vi "side_ir_microstep.vi"(0 "IN-OUT":enum16{"out", "in"}(ring), 1 "IR_L":dbl, 2 "IR_R":dbl, 5 "Step":i32, 7 "Stop Mode":string(combo), 9 "Delay":i32, 11 "logic_num":dbl, 12 "Zeta_B":i32, 13 "Zeta_F":i32) -> (4 "OZeta_b":i32, 6 "Ozeta_f":i32, 8 "Done":bool)   [LabVIEW 2017]
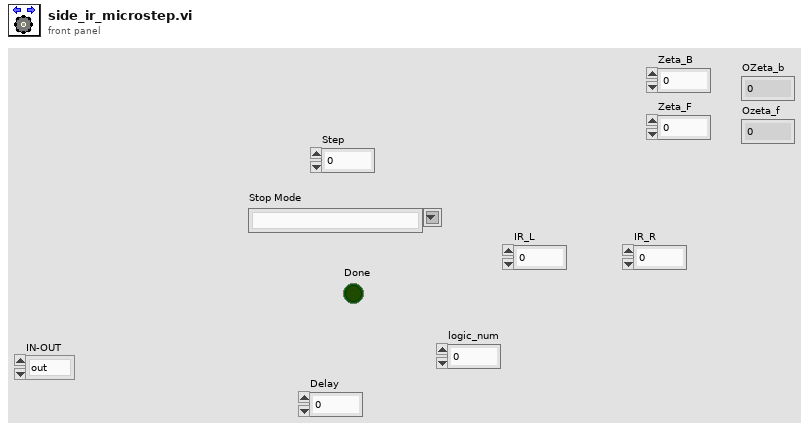
[diagram p1: front panel]
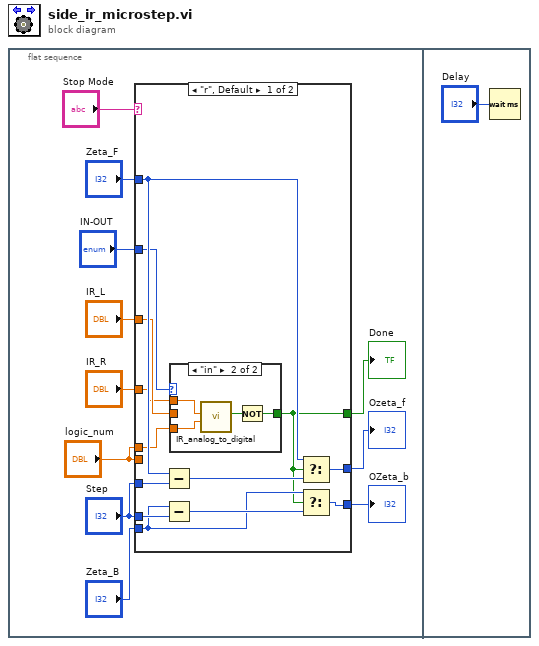
[diagram p0: block diagram]
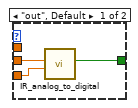
[diagram p2: hidden frame]
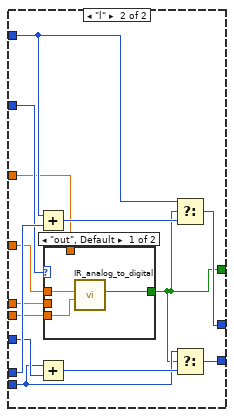
[diagram p3: hidden frame]
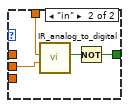
[diagram p4: hidden frame]
diagram:
  n1 = flat-sequence {
    frame #0 {
      n2 = case shown="\"r\", Default" "Stop Mode" {
        tunnel: "IR_L" -> [w15 w32]
        tunnel: "logic_num" -> [w14 w34]
        tunnel: [w19 w44] -> w5
        tunnel: [w20 w43] -> w4
        tunnel: [w13 w33] -> w9
        tunnel: "Zeta_B" -> [w18 w39]
        tunnel: "Zeta_F" -> [w17 w38]
        tunnel: "Step" -> [w21 w41]
        tunnel: "Step" -> [w22 w40]
        tunnel: "IN-OUT" -> [w16 w37]
        tunnel: "logic_num" -> [_ w36]
        tunnel: "IR_R" -> [w12 w35]
        frame "r", Default {
          n3 = Subtract(x=w17, y=w22) -> (x-y=w24:i32)
          n4 = Subtract(x=w18, y=w21) -> (x-y=w23:i32)
          n5 = case shown="\"in\"" w16 {
            tunnel: [w27 w30] -> w13
            tunnel: w15 -> [w26 _]
            tunnel: w14 -> [w25 w29]
            tunnel: w12 -> [_ w28]
            frame "out", Default {
              n6 = call "IR_analog_to_digital.vi"("logic_num"=w25, "IR_IN"=w26) -> ("IR_OUT"=w27:bool)  [unwired: 9 in]
            }
            frame "in" {
              n7 = call "IR_analog_to_digital.vi"("logic_num"=w29, "IR_IN"=w28) -> ("IR_OUT"=w31:bool)  [unwired: 9 in]
              n8 = Not(x=w31) -> (.not. x?=w30:bool)
            }
          }
          n9 = Select(t=w17, s=w13, f=w24) -> (s? t:f=w19:i32)
          n10 = Select(t=w18, s=w13, f=w23) -> (s? t:f=w20:i32)
        }
        frame "l" {
          n11 = Add(x=w38, y=w41) -> (x+y=w45:i32)
          n12 = Add(x=w39, y=w40) -> (x+y=w42:i32)
          n13 = case shown="\"out\", Default" w37 {
            tunnel: w36 -> [w48 _]
            tunnel: w35 -> [w47 _]
            tunnel: [w46 w50] -> w33
            tunnel: w34 -> [_ w52]
            tunnel: w32 -> [_ w49]
            frame "out", Default {
              n14 = call "IR_analog_to_digital.vi"("logic_num"=w48, "IR_IN"=w47) -> ("IR_OUT"=w46:bool)  [unwired: 9 in]
            }
            frame "in" {
              n15 = call "IR_analog_to_digital.vi"("logic_num"=w52, "IR_IN"=w49) -> ("IR_OUT"=w51:bool)  [unwired: 9 in]
              n16 = Not(x=w51) -> (.not. x?=w50:bool)
            }
          }
          n17 = Select(t=w38, s=w33, f=w45) -> (s? t:f=w44:i32)
          n18 = Select(t=w39, s=w33, f=w42) -> (s? t:f=w43:i32)
        }
      }
      "OZeta_b" <- w4
      "Ozeta_f" <- w5
      "Done" <- w9
    }
    frame #1 {
      n19 = Wait (ms)(milliseconds to wait="Delay") -> ()  [unwired: 1 out]
    }
  }
